vi "NovaTech409A_FreqPow.vi"(0 "VISA resource name":refnum<visa-resource-name>="COM1", 1 "Freq":dbl, 2 "Power":u16, 3 "error in (no error)":errorcluster, 4 "Channel (0-3)":u8 max=3) -> (5 "VISA resource name out":refnum<visa-resource-name>="COM1", 6 "error out":errorcluster)   [LabVIEW 2013, in "Novatech 409A.lvlib"]
uses:
  Novatech 409A.lvlib
panel:
  out "resulting string 2":string
  out "resulting string":string
  out "read buffer 2":string
  out "read buffer 1":string
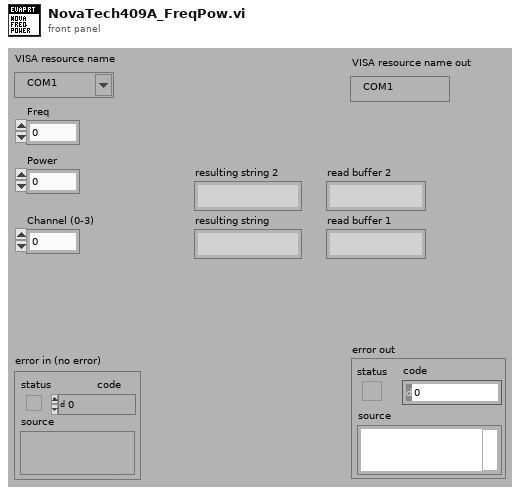
[diagram p1: front panel]
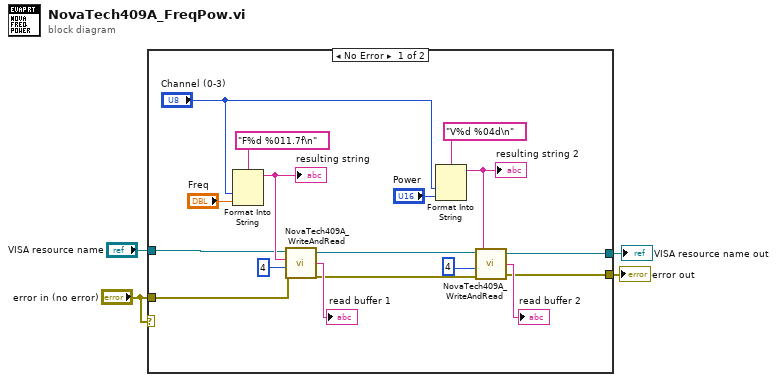
[diagram p0: block diagram]
diagram:
  n1 = case shown="No Error" "error in (no error)" {
    tunnel: "VISA resource name" -> [w16 w22]
    tunnel: "error in (no error)" -> [w15 w23]
    tunnel: [w9 w22] -> w3
    tunnel: [w8 w23] -> w2
    frame No Error {
      n2 = Format Into String(format string="F%d %011.7f\n", "Channel (0-3)", "Freq") -> (resulting string=w17:string)  [unwired: 2 in, 1 out]
      "resulting string" <- w17
      n3 = call "NovaTech409A_WriteAndRead.vi"("error in (no error)"=w15, "Number of Bytes"=4, "write buffer"=w17, "VISA resource name"=w16) -> ("error out"=w11:errorcluster, "read buffer"=→"read buffer 1":string, "VISA resource name out"=w12:refnum<visa-resource-name>)
      n4 = Format Into String(format string="V%d %04d\n", "Channel (0-3)", "Power") -> (resulting string=w13:string)  [unwired: 2 in, 1 out]
      "resulting string 2" <- w13
      n5 = call "NovaTech409A_WriteAndRead.vi"("error in (no error)"=w11, "Number of Bytes"=4, "write buffer"=w13, "VISA resource name"=w12) -> ("error out"=w8:errorcluster, "read buffer"=→"read buffer 2":string, "VISA resource name out"=w9:refnum<visa-resource-name>)
    }
    frame Error {
    }
  }
  "error out" <- w2
  "VISA resource name out" <- w3
